vi "Extract Numbers with Match Pattern.vi"() -> ()   [LabVIEW 2023]
doc: "Uses the Match Pattern function to find all numbers in the given string, and returns them in an array. All of the following formats are recognized:\n\n123 1.23 .123 0.123 -1.23\n\nNo spaces or other characters may appear within the number, but any characters may appear before or after the number. This example assumes that the input string contains periods and not commas for the decimal separator."
panel:
  out "Extracted Numbers":dbl[](array[numeric]) format="%#.6g"
  in  "String":string="one 2 -3 4.0 5.5"
  # "Overview: Demonstrates how to use the Match Pattern function to extract numeric values from a string.\nInstructions:\n1. Specify a String value containing numbers.\n2. Run the VI. All numbers in the String are displayed in the Extracted Numbers array."
  # "Note: Numbers that are spelled out (like \"one\" in the string above) are not interpreted as numbers.  Scientific notation is also not handled by this example. Additionally, this example will only extract decimal numbers from the string that use the \".\" character as a decimal separator."
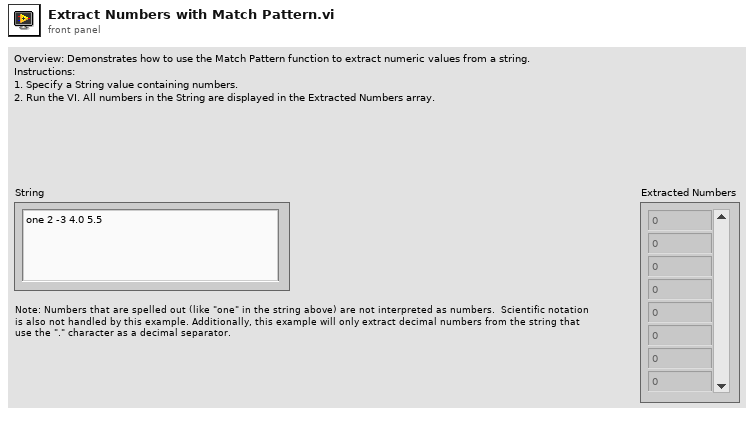
[diagram p1: front panel]
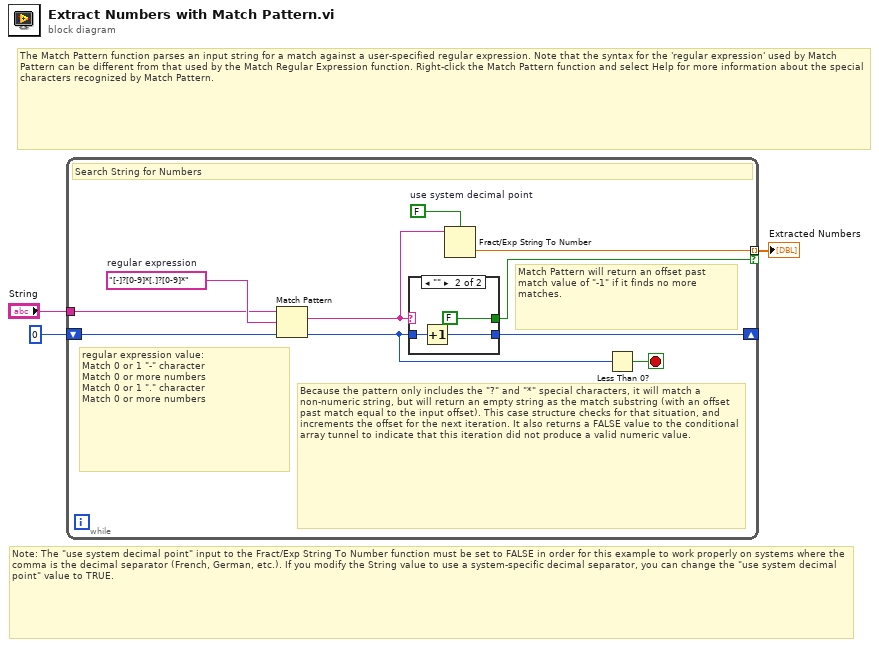
[diagram p0: block diagram]
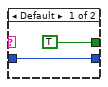
[diagram p2: hidden frame]
diagram:
  # "Note: The \"use system decimal point\" input to the Fract/Exp String To Number function must be set to FALSE in order for this example to work properly on systems where the comma is the decimal separator (French, German, etc.). If you modify the String value to use a system-specific decimal separator, you can change the \"use system decimal point\" value to TRUE."
  # "The Match Pattern function parses an input string for a match against a user-specified regular expression. Note that the syntax for the 'regular expression' used by Match Pattern can be different from that used by the Match Regular Expression function. Right-click the Match Pattern function and select Help for more information about the special characters recognized by Match Pattern."
  n1 = while {
    shift-left: 0 -> [w9]
    shift-right: [w4] -> _
    tunnel: [w13] -> w3 mode=indexing if=w6
    tunnel: "String" -> [w8]
    stop <- w12 stop-if-true
    w11 = FALSE  # use system decimal point
    w10 = "[-]?[0-9]*[.]?[0-9]*"  # regular expression
    # "Match Pattern will return an offset past match value of \"-1\" if it finds no more matches."
    # "Because the pattern only includes the \"?\" and \"*\" special characters, it will match a non-numeric string, but will return an empty string as the match substring (with an offset past match equal to the input offset). This case structure checks for that situation, and increments the offset for the next iteration. It also returns a FALSE value to the conditional array tunnel to indicate that this iteration did not produce a valid numeric value."
    # "regular expression value:\nMatch 0 or 1 \"-\" character\nMatch 0 or more numbers\nMatch 0 or 1 \".\" character\nMatch 0 or more numbers"
    # "Search String for Numbers"
    n2 = Match Pattern(string=w8, regular expression=w10, offset (0)=w9) -> (match substring=w7:string, offset past match=w5:i32)  [unwired: 2 out]
    n3 = case shown="\"\"" w7 {
      tunnel: [w15 w17] -> w4
      tunnel: [TRUE FALSE] -> w6
      tunnel: w5 -> [w15 w18]
      frame Default {
      }
      frame "" {
        n4 = Increment(x=w18) -> (x+1=w17:i32)
      }
    }
    n5 = Fract/Exp String To Number(use system decimal point (T)=w11, string=w7) -> (number=w13:dbl)  [unwired: 2 in, 1 out]
    n6 = Less Than 0?(x=w5) -> (x < 0?=w12:bool)
  }
  "Extracted Numbers" <- w3
